vi "ULx Read (Composite 1DWfm NChan NSamp).vi"(0 "task in":refnum<k24>, 7 "number of samples per channel":i32=-1, 9 "timeout":dbl=10.0 format="%_4g", 11 "error in":errorcluster) -> (4 "task out":refnum<k24>, 6 "analog data":waveform(dbl)[](array[waveform]), 8 "digital data":digitalwaveform[](array[waveform]), 10 "counter data":waveform(dbl)[](array[waveform]), 15 "error out":errorcluster)   [LabVIEW 2020]
doc: "Reads one or more waveforms from a task that contains one or more composite input channels."
uses:
  C:/Users/William/Documents/LV 2020 builds/LeaktestDAQ/Source-v33/ULx_LV.dll
  ULx_LV.dll
panel:
  # "channel"
  # "channel"
  # "sample #"
  # "channel"
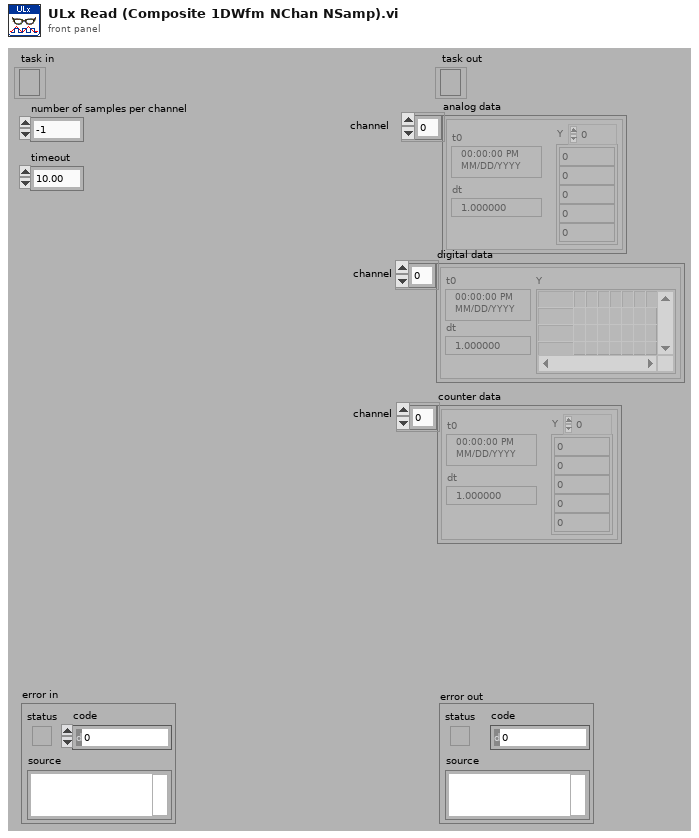
[diagram p1: front panel]
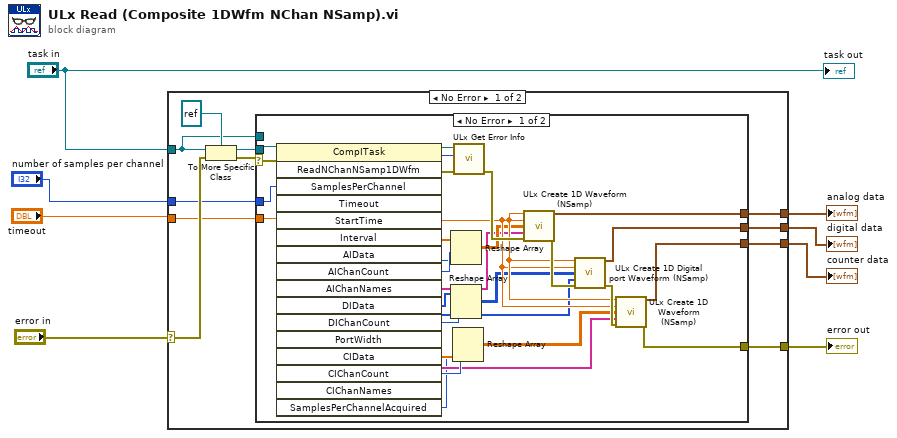
[diagram p0: block diagram]
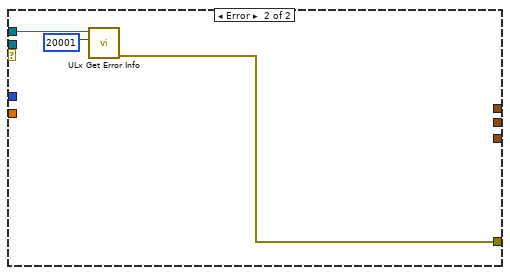
[diagram p2: hidden frame]
diagram:
  n1 = case shown="No Error" "error in" {
    selector: "error in" -> [w19 w52]
    tunnel: "task in" -> [w11 _]
    tunnel: "timeout" -> [w15 _]
    tunnel: [w12 _] -> w3
    tunnel: [w14 w52] -> w6
    tunnel: "number of samples per channel" -> [w13 _]
    tunnel: [w10 _] -> w1
    tunnel: [w9 _] -> w2
    frame No Error {
      n2 = To More Specific Class(target class=refnum<k24> refnum, reference=w11, error in=w19) -> (specific class reference=w16:refnum<k24>, error out=w17:errorcluster)
      n3 = case shown="No Error" w17 {
        selector: w17 -> [w47 _]
        tunnel: w16 -> [w48 _]
        tunnel: w15 -> [w44 _]
        tunnel: [w33 w49] -> w14
        tunnel: w13 -> [w43 _]
        tunnel: [w41 _] -> w12
        tunnel: w11 -> [_ w51]
        tunnel: [w37 _] -> w10
        tunnel: [w36 _] -> w9
        frame No Error {
          n4 = invoke class="CompITask" method="ReadNChanNSamp1DWfm"(reference=w48, error in=w47, "SamplesPerChannel"=w43, "Timeout"=w44) -> (reference out=w45:refnum<k24>, error out=w46:errorcluster, "ReadNChanNSamp1DWfm"=w42:i32, "StartTime"=w35:dbl, "Interval"=w34:dbl, "AIData"=w32:dbl[], "AIChanCount"=w31:i32, "AIChanNames"=w29:string[], "DIData"=w28:u32[], "DIChanCount"=w27:i32, "PortWidth"=w25:i32[], "CIData"=w24:dbl[], "CIChanCount"=w23:i32, "CIChanNames"=w22:string[], "SamplesPerChannelAcquired"=w21:i32)  [unwired: 13 in, 2 out]
          n5 = Reshape Array(w32, w31, w21) -> (w30:dbl[][])
          n6 = Reshape Array(w28, w27, w21) -> (w26:u32[][])
          n7 = Reshape Array(w24, w23, w21) -> (w20:dbl[][])
          n8 = call "ULx Get Error Info.vi"("error in"=w46, "ErrorCode"=w42, "task in"=w45) -> ("error out"=w40:errorcluster)  [unwired: 8 in]
          n9 = call "ULx Create 1D Waveform (NSamp).vi"("t0"=w35, "dt"=w34, "data Array"=w30, "channelName Array"=w29, "error in"=w40) -> ("data"=w41:waveform(dbl)[], "error out"=w39:errorcluster)  [unwired: 9 in]
          n10 = call "ULx Create 1D Digital port Waveform (NSamp).vi"("t0"=w35, "dt"=w34, "data Array"=w26, "port widths"=w25, "error in"=w39) -> ("data"=w36:digitalwaveform[], "error out"=w38:errorcluster)  [unwired: 9 in]
          n11 = call "ULx Create 1D Waveform (NSamp).vi"("t0"=w35, "dt"=w34, "data Array"=w20, "channelName Array"=w22, "error in"=w38) -> ("data"=w37:waveform(dbl)[], "error out"=w33:errorcluster)  [unwired: 9 in]
        }
        frame Error {
          n12 = call "ULx Get Error Info.vi"("ErrorCode"=20001, "task in"=w51) -> ("error out"=w49:errorcluster)  [unwired: 9 in]
        }
      }
    }
    frame Error {
    }
  }
  "error out" <- w6
  "analog data" <- w3
  "digital data" <- w2
  "counter data" <- w1
  "task out" <- "task in"
